vi "Sequences folder.vi"(11 "error in (no error)":errorcluster) -> (8 "Sequence folder":path, 15 "error out":errorcluster)   [LabVIEW 2011]
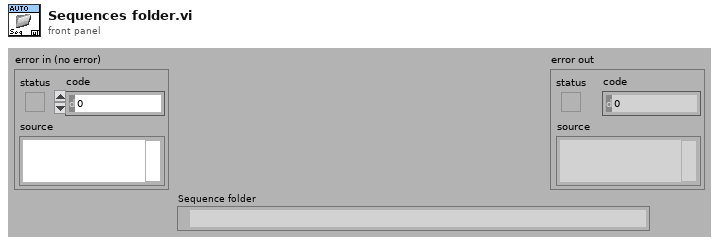
[diagram p1: front panel]
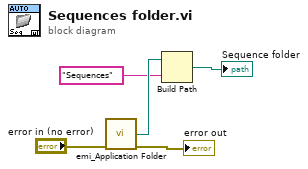
[diagram p0: block diagram]
diagram:
  n1 = call "emi_Application Folder.vi"("error in (no error)"="error in (no error)") -> ("Dir"=w5:path, "error out"=→"error out":errorcluster)  [unwired: 13 in]
  n2 = Build Path(base path=w5, name or relative path="Sequences") -> (appended path=→"Sequence folder":path)
